vi "Create Master Instance.vi"   [LabVIEW 2018, in "Modbus Master.lvclass"]
doc: "Creates a serial or TCP Modbus master instance. You must manually select the polymorphic instance to use."
uses:
  Modbus Master.lvclass
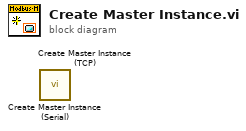
[diagram p0: block diagram]
diagram:
  n1 = call "Create Master Instance (Serial).vi"() -> ()  [unwired: 10 in, 2 out]
  n2 = call "Create Master Instance (TCP).vi"() -> ()  [unwired: 10 in, 2 out]
